vi "PIZApproaching.vi"() -> ()   [LabVIEW 2014]
uses:
  <vilib>/rvi/Emulation/niFpgaSctlEmulationGetInTimedLoop.vi
  <vilib>/rvi/eio/common/nirviEmuTemplateMethod_errors.vi
  <vilib>/rvi/Emulation/niFpgaProcessEmulError.vi
  <vilib>/rvi/Emulation/niFpgaGetClockAttributes.vi
  <vilib>/rvi/Emulation/niFpgaEmulationReportErrorSimple.vi
  <vilib>/rvi/Emulation/niFpgaCriticalErrorInLSC.vi
  <vilib>/eio/EIONode/EIONode.xnode
panel:
  in  "stepMultiplier / 0.305nm":i16
  in  "thresholdIndex":i16
  out "preCurrIndex":i16
  out "refCurrIndex":i16
  out "NotApproached?":bool
  out "PIZPos":i16
  in  "stop":bool
  out "Approached?":bool
  in  "Sleep ms":i16
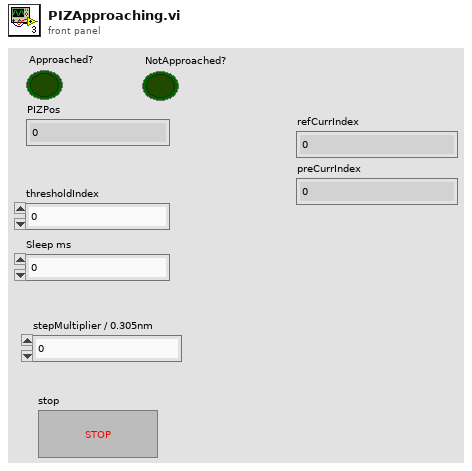
[diagram p1: front panel]
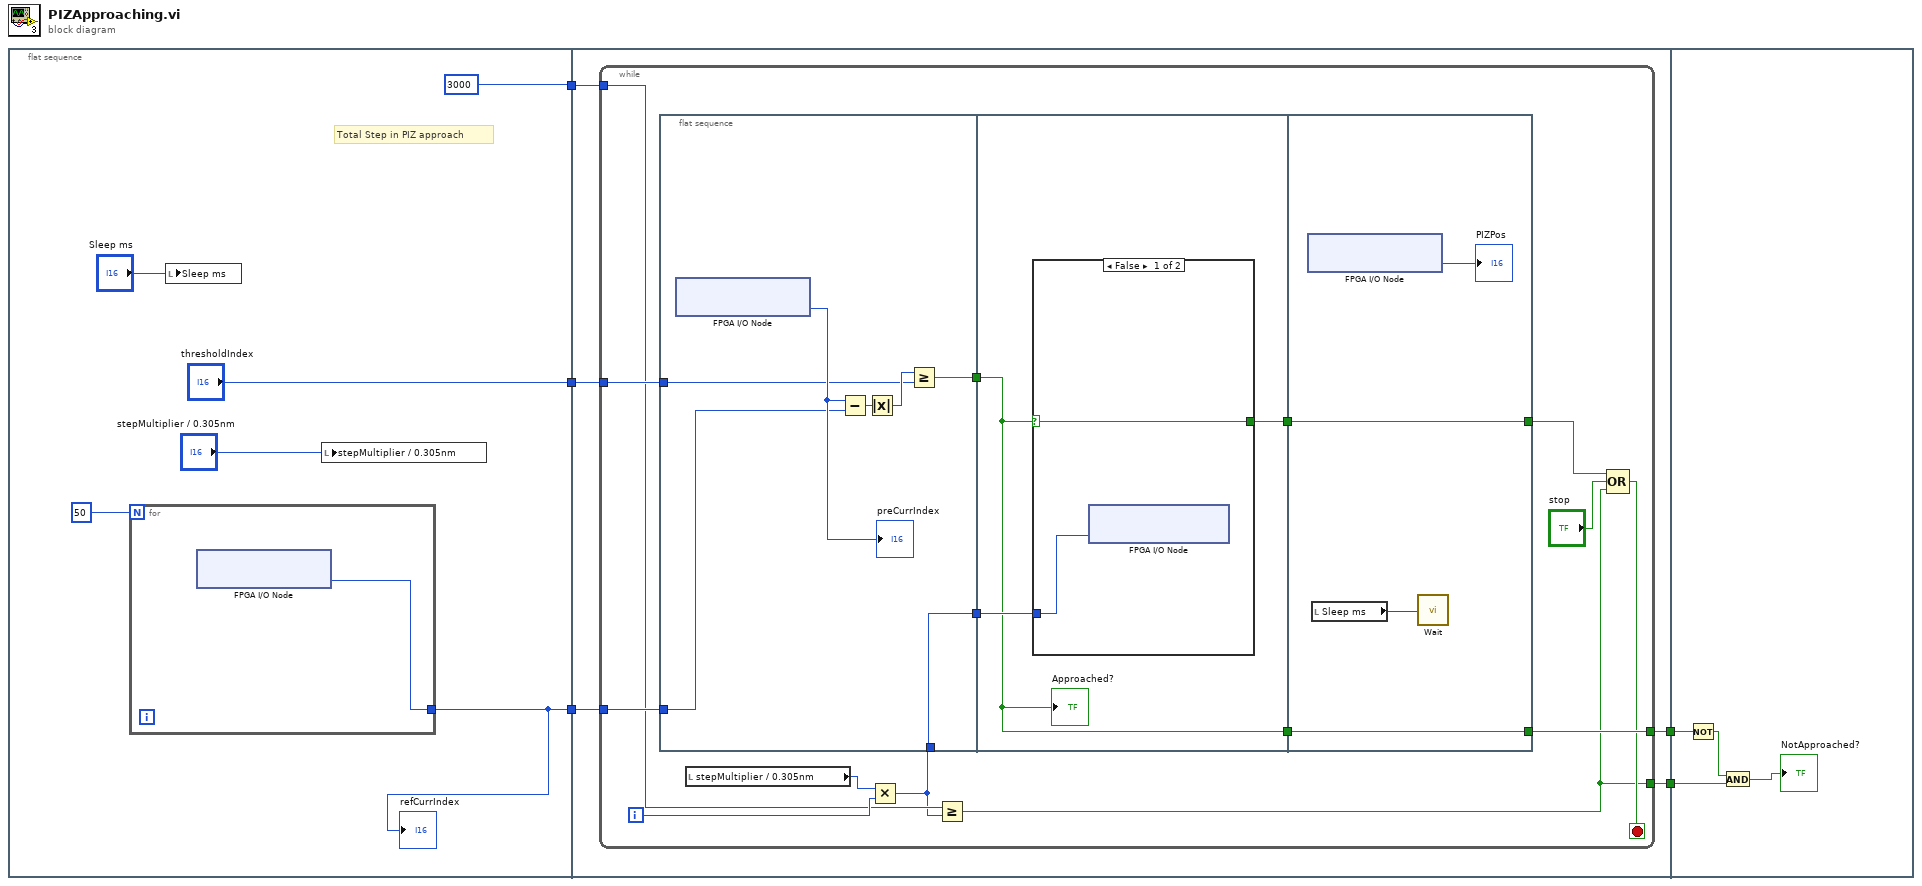
[diagram p0: block diagram]
diagram:
  n1 = flat-sequence {
    tunnel: [i16 3000] -> w5
    tunnel: [w7] -> w4
    tunnel: ["thresholdIndex"] -> w3
    tunnel: w5 -> [w14]
    tunnel: w4 -> [w16]
    tunnel: w3 -> [w17]
    tunnel: [w15] -> w2
    tunnel: [w13] -> w1
    tunnel: w2 -> [w53]
    tunnel: w1 -> [w50]
    frame #0 {
      # "Total Step in PIZ approach"
      n2 = for {
        N: 50 -> [_]
        tunnel: [w12] -> w7
        n3 = xnode "FPGA I/O Node"() -> ("Connector0/AI1"=w12:i16)  [unwired: 1 in, 1 out]
      }
      "refCurrIndex" <- w7
      n4 = local write "Sleep ms"("Sleep ms") -> ()
      n5 = local write "stepMultiplier / 0.305nm"("stepMultiplier / 0.305nm") -> ()
    }
    frame #1 {
      n6 = while {
        tunnel: w17 -> [w31]
        tunnel: w16 -> [w32]
        tunnel: [w28] -> w15
        tunnel: w14 -> [w20]
        tunnel: [w18] -> w13
        i -> [w21]
        stop <- w23 stop-if-true
        n7 = flat-sequence {
          tunnel: w32 -> [w38]
          tunnel: w31 -> [w35]
          tunnel: [w34] -> w30
          tunnel: [w33] -> w29
          tunnel: w19 -> [w33]
          tunnel: w29 -> [w41]
          tunnel: w30 -> [w40]
          tunnel: [w42] -> w27
          tunnel: [w40] -> w26
          tunnel: [w48] -> w28
          tunnel: [w49] -> w25
          tunnel: w27 -> [w49]
          tunnel: w26 -> [w48]
          frame #0 {
            n8 = xnode "FPGA I/O Node"() -> ("Connector0/AI1"=w39:i16)  [unwired: 1 in, 1 out]
            "preCurrIndex" <- w39
            n9 = Subtract(x=w39, y=w38) -> (x-y=w37:i16)
            n10 = Absolute Value(x=w37) -> (abs(x)=w36:i16)
            n11 = Greater Or Equal?(x=w36, y=w35) -> (x >= y?=w34:bool)
          }
          frame #1 {
            n12 = case shown="False" w40 {
              selector: w40 -> [w44 w45]
              tunnel: [w44 w45] -> w42
              tunnel: w41 -> [w43 _]
              frame False {
                n13 = xnode "FPGA I/O Node"("Connector0/AO0"=w43) -> ()  [unwired: 1 in, 1 out]
              }
              frame True {
              }
            }
            "Approached?" <- w40
          }
          frame #2 {
            n14 = xnode "FPGA I/O Node"() -> ("Connector0/AI0"=→"PIZPos":i16)  [unwired: 1 in, 1 out]
            n15 = local read "Sleep ms"() -> (w47:i16)
            n16 = call "Wait"("Count(mSec)"=w47) -> ()  [unwired: 1 out]
          }
        }
        n17 = local read "stepMultiplier / 0.305nm"() -> (w22:i16)
        n18 = Multiply(x=w22, y=w21) -> (x*y=w19:i32)
        n19 = Greater Or Equal?(x=w20, y=w19) -> (x >= y?=w18:bool)
        n20 = Compound Arithmetic op=OR(w25, "stop", w18) -> (w23:bool)
      }
    }
    frame #2 {
      n21 = Not(x=w53) -> (.not. x?=w52:bool)
      n22 = And(x=w52, y=w50) -> (x .and. y?=→"NotApproached?":bool)
    }
  }
